vi "Open FPGA Ref_No Run.vi"(8 "error in (no error)":errorcluster, 10 "resource name":string, 11 "starter kit host 2.0 in":refnum<class "NI_Robotics_Starter Kit Host_9632_2.0.lvclass">) -> (0 "error out":errorcluster, 2 "FPGA Interface":T1, 3 "starter kit host 2.0 out":refnum<class "NI_Robotics_Starter Kit Host_9632_2.0.lvclass">)   [LabVIEW 2017, in "NI_Robotics_Starter Kit Host_9632_2.0.lvclass"]
uses:
  <vilib>/robotics/Starter Kit/2.0/9632 Host Interface/NI_Robotics_Starter Kit Host_9632_2.0.lvclass
  <vilib>/robotics/Starter Kit/2.0/FPGA Host Interface/FPGA Refnum.ctl
  <vilib>/rvi/interface/common/dynamic/niFpgaDynamicAddResources.vi
  <vilib>/FPGAPlugInAG/sbRIO-9632/niLvFpga_Open_sbRIO-9632.vi
  <vilib>/rvi/interface/nirviOpenFPGA/nirviOpenFPGA.xnode
  <vilib>/robotics/Starter Kit/FPGA Bitfiles/Starter Kit 2.0_9632.lvbitx
  <vilib>/robotics/Starter Kit/2.0/FPGA Host Interface/NI_Robotics_Starter Kit Host_FPGA_2.0.lvclass
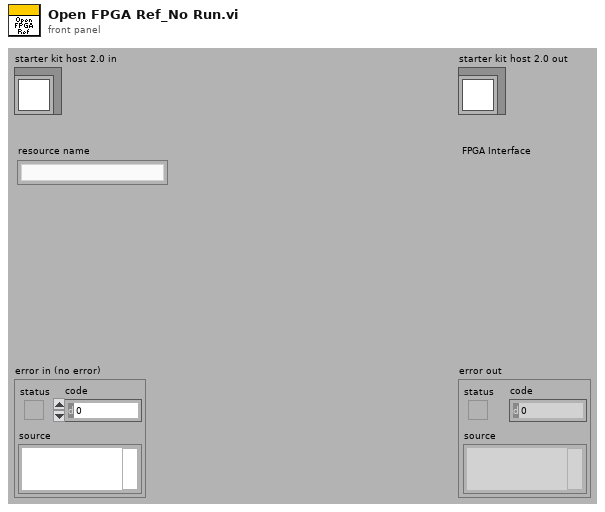
[diagram p1: front panel]
types:
  T1 = typedef "NI_Robotics_Starter Kit Host_FPGA_2.0.lvclass/FPGA Refnum.ctl" = refnum<k20>
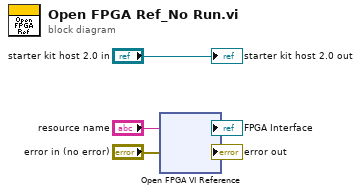
[diagram p0: block diagram]
diagram:
  n1 = xnode "Open FPGA VI Reference"("error in"="error in (no error)", "resource name"="resource name") -> ("FPGA VI Reference Out"=→"FPGA Interface":refnum<k20>, "error out"=→"error out":errorcluster)
  "starter kit host 2.0 out" <- "starter kit host 2.0 in"
